vi "Database-NewData.vi"(8 "error in":errorcluster, 10 "Data":T1 {"Values" format="%.3f"}, 11 "Idx":i32) -> (0 "error out":errorcluster, 2 "Saved":bool)   [LabVIEW 2016]
doc: "Go to DB->WriteStationValues action\nReturn boolean flag to show if data was saved to DB successfully\n\nWabco 2017 All right reserved\nAuthor: maciej.szupienko@wabco-auto.com"
uses:
  Drivers/PLC/LowLevel/PLC.DataBlock.PLCvalues.ctl
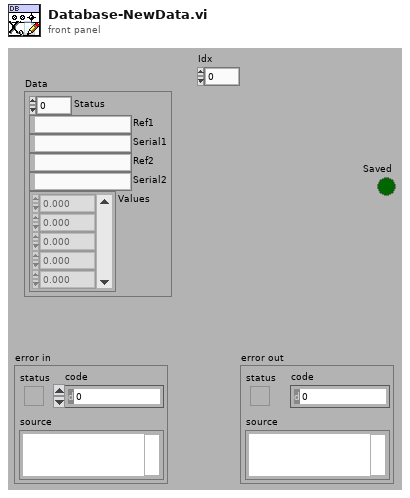
[diagram p1: front panel]
types:
  T1 = typedef "PLC.DataBlock.PLCvalues.ctl" = cluster{"Status":u8, "Ref1":string, "Serial1":string, "Ref2":string, "Serial2":string, "Values":sgl[]}
  T2 = typedef "Database.Data.Sets.ctl" = cluster{"Enable":bool, "ConnString":string, "SystemName":string, "CheckExistSystems":string[], "PrevSystems":string[]}
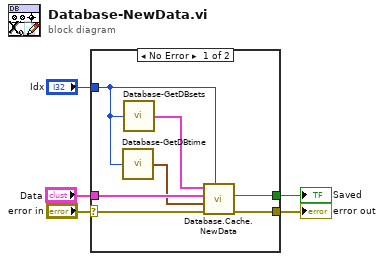
[diagram p0: block diagram]
diagram:
  n1 = case shown="No Error" "error in" {
    selector: "error in" -> [w12 w13]
    tunnel: [w11 w13] -> w4
    tunnel: "Data" -> [w10 _]
    tunnel: "Idx" -> [w8 _]
    tunnel: [w6 _] -> w1
    frame No Error {
      n2 = call "Database-GetDBtime.vi"("Idx"=w8) -> ("DbTime"=w9:timestamp)
      n3 = call "Database-GetDBsets.vi"("Idx"=w8) -> ("Sets"=w7:T2)
      n4 = call "Database.Cache.NewData.vi"("Idx"=w8, "error in"=w12, "DBtime"=w9, "Data"=w10, "Sets"=w7) -> ("error out"=w11:errorcluster, "Data saved"=w6:bool)  [unwired: 5 in]
    }
    frame Error {
    }
  }
  "error out" <- w4
  "Saved" <- w1
